vi "signal_generation_0.vi"() -> ()   [LabVIEW 2016]
uses:
  controls/State.ctl
  <vilib>/Utility/error.llb/DialogType.ctl
  <vilib>/DAQmx/write.llb/DAQmx Write (Analog Wfm 1Chan NSamp).vi
  <vilib>/DAQmx/write.llb/DAQmx Write (Analog DBL 1Chan 1Samp).vi
  <vilib>/DAQmx/read.llb/DAQmx Read (Analog 1D Wfm NChan NSamp).vi
  <vilib>/DAQmx/create/channels.llb/DAQmx Create Channel (AO-Voltage-Basic).vi
  <vilib>/DAQmx/create/channels.llb/DAQmx Create Channel (AI-Voltage-Basic).vi
  <vilib>/DAQmx/configure/timing.llb/DAQmx Timing (Sample Clock).vi
  <vilib>/DAQmx/miscellaneous.llb/DAQmx Fill In Error Info.vi
  <resource>/objmgr/daqmx.rc
  <vilib>/measure/NI_MABase.lvlib
panel:
  out "Waveform Graph 2":waveform(dbl)[](graph)=[{"t0"=timestamp(3594732894.3389087 s since 1904-01-01), "dt"=0.001, "Y"=array[1000 elements], "attributes"=variant("NI_ChannelName"=variant(string "DAQ_6363/ai0"), "NI_UnitDescription"=variant(string "Volts"))}]
  in  "DAQ channel 3 In":tag="DAQ_6363/ai0"
  out "error out":errorcluster
  in  "Number of Samples":i32=1000
  in  "Samples per Period":dbl=100.0
  in  "DAQ channel 2 In":tag="DAQ_6363/ao1"
  in  "DAQ channel 1 In":tag="DAQ_6363/ao0"
  in  "Error In (no error)":errorcluster
  in  "Exit Button":bool
  out "Status":string="Off"
  in  "TMA Voltage On/Off":bool
  in  "Sawtooth Signal On/Off":bool
  out "Waveform Graph":waveform(dbl)(graph)={"t0"=timestamp(0 s since 1904-01-01), "dt"=0.001, "Y"=array[1000 elements]}
  in  "TMA Voltage":dbl=2.0 min=-10.0 max=10.0
  in  "Period (ms)":dbl=100.0 min=0.01
  in  "Amplitude (V)":dbl=2.0 min=0.0 max=30.0
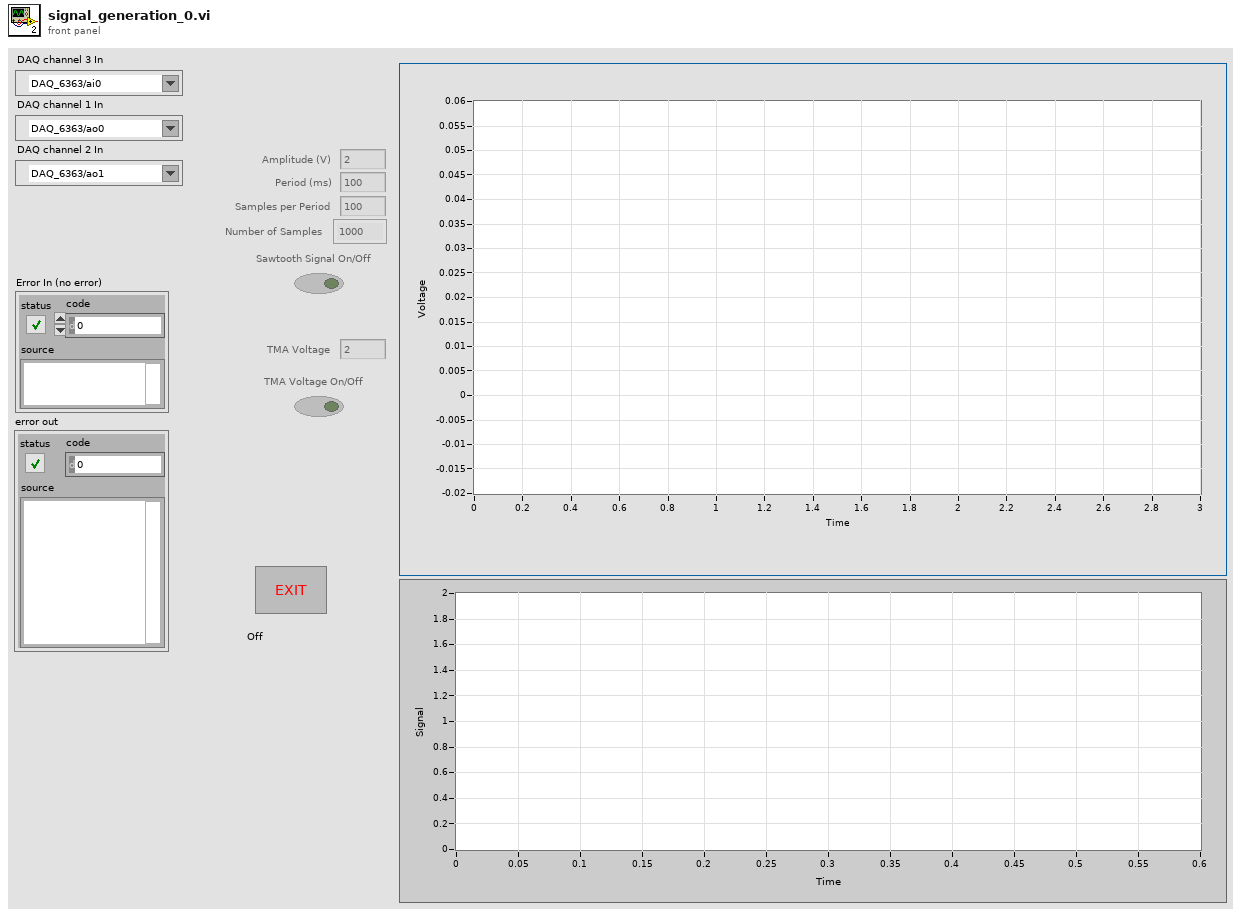
[diagram p1: front panel]
types:
  T1 = typedef "State.ctl" = enum16{"Init", "Idle", "Shutdown"}
  T2 = enum16{"Sine Wave", "Triangle Wave", "Square Wave", "Sawtooth Wave"}
  T3 = typedef "DialogType.ctl" = u16
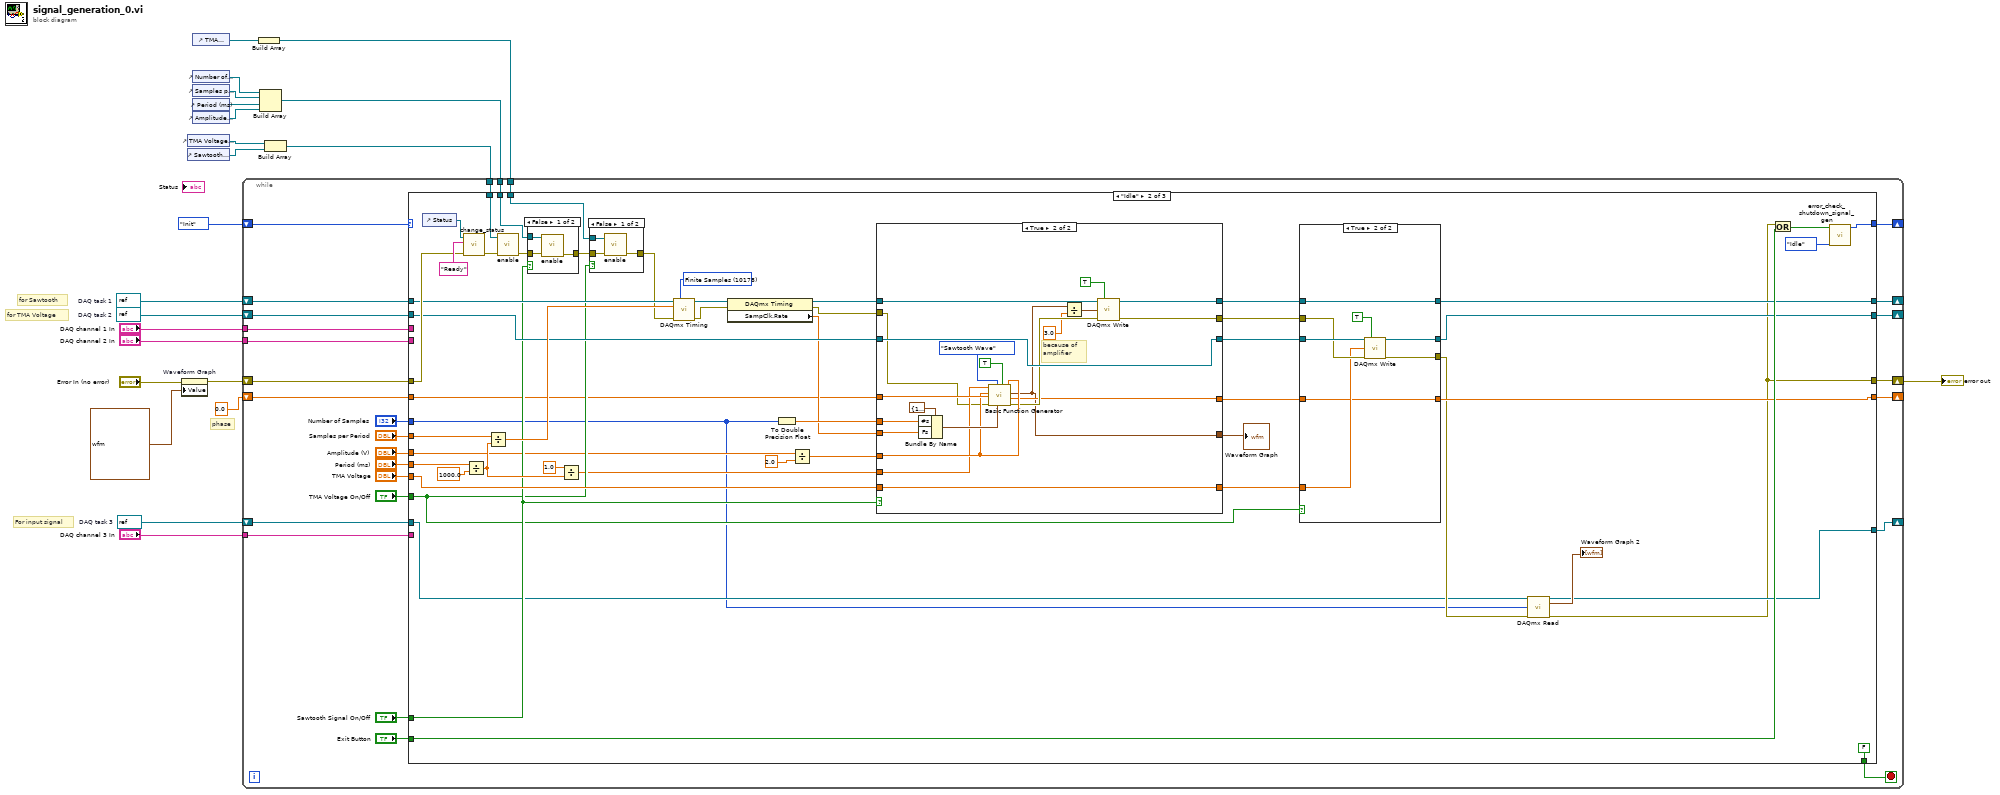
[diagram p0: block diagram]
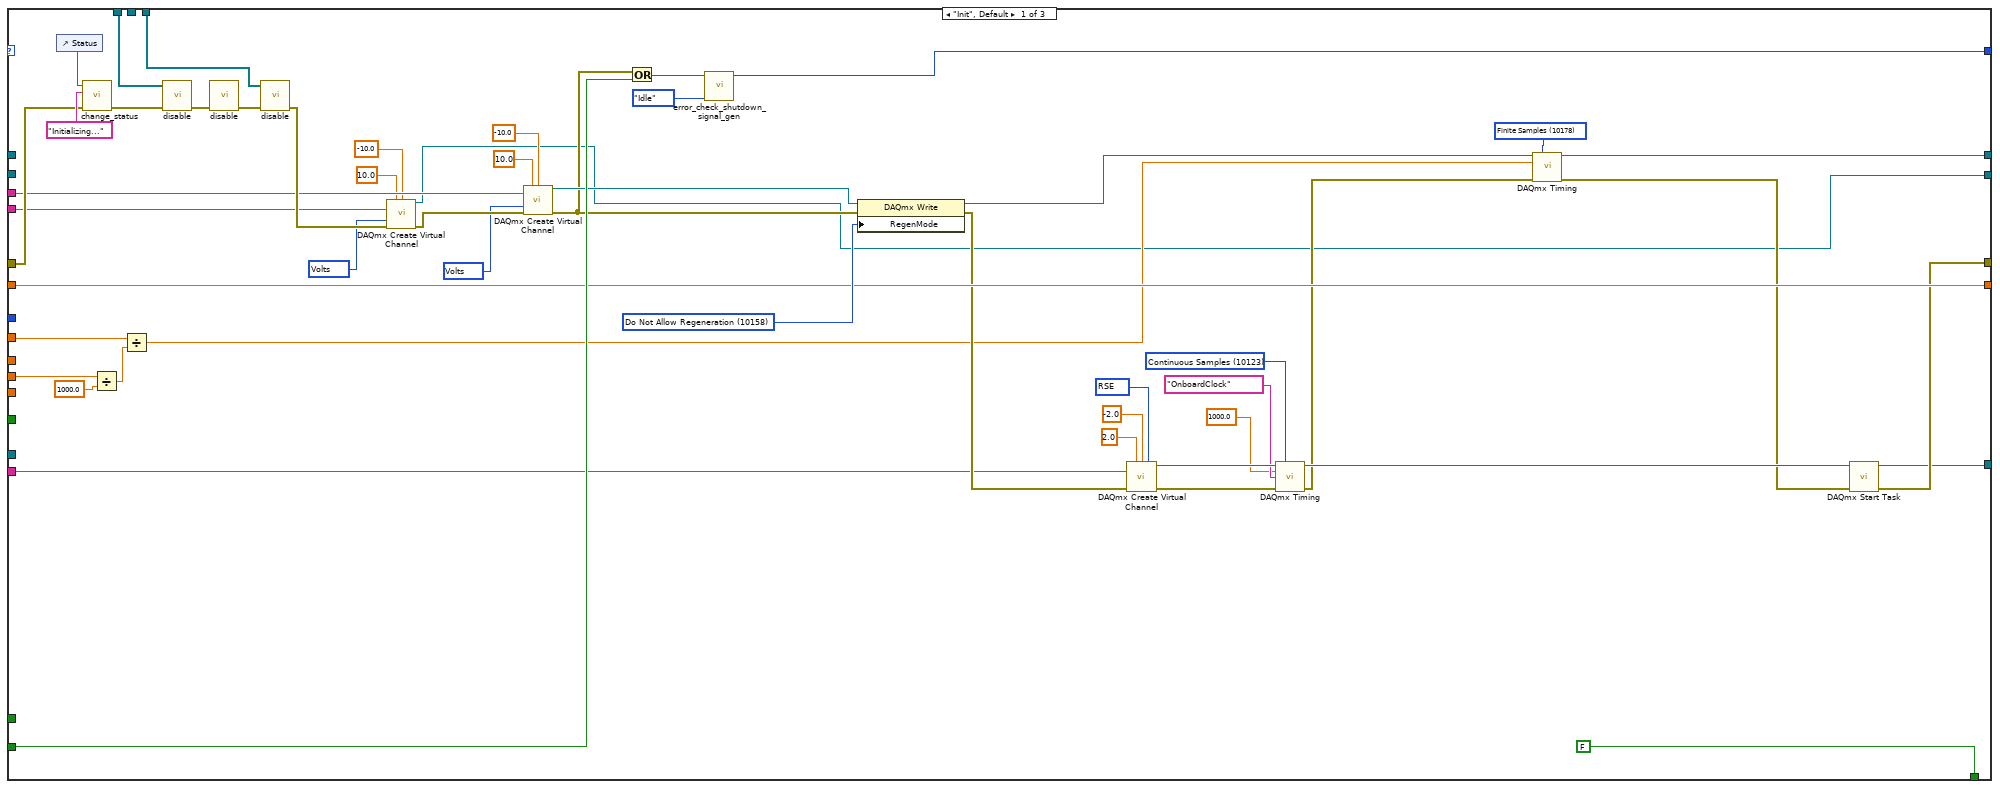
[diagram p2: hidden frame]
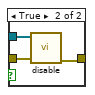
[diagram p3: hidden frame]
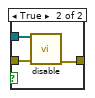
[diagram p4: hidden frame]
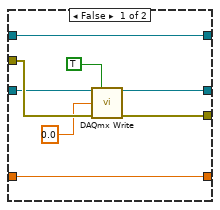
[diagram p5: hidden frame]
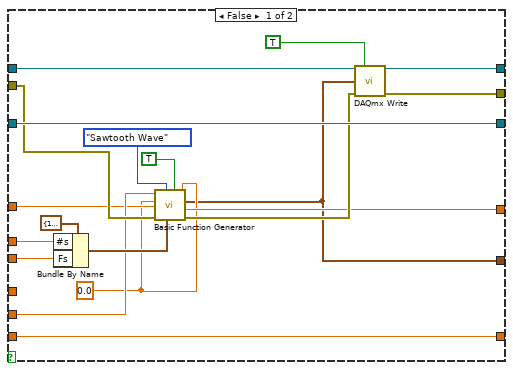
[diagram p6: hidden frame]
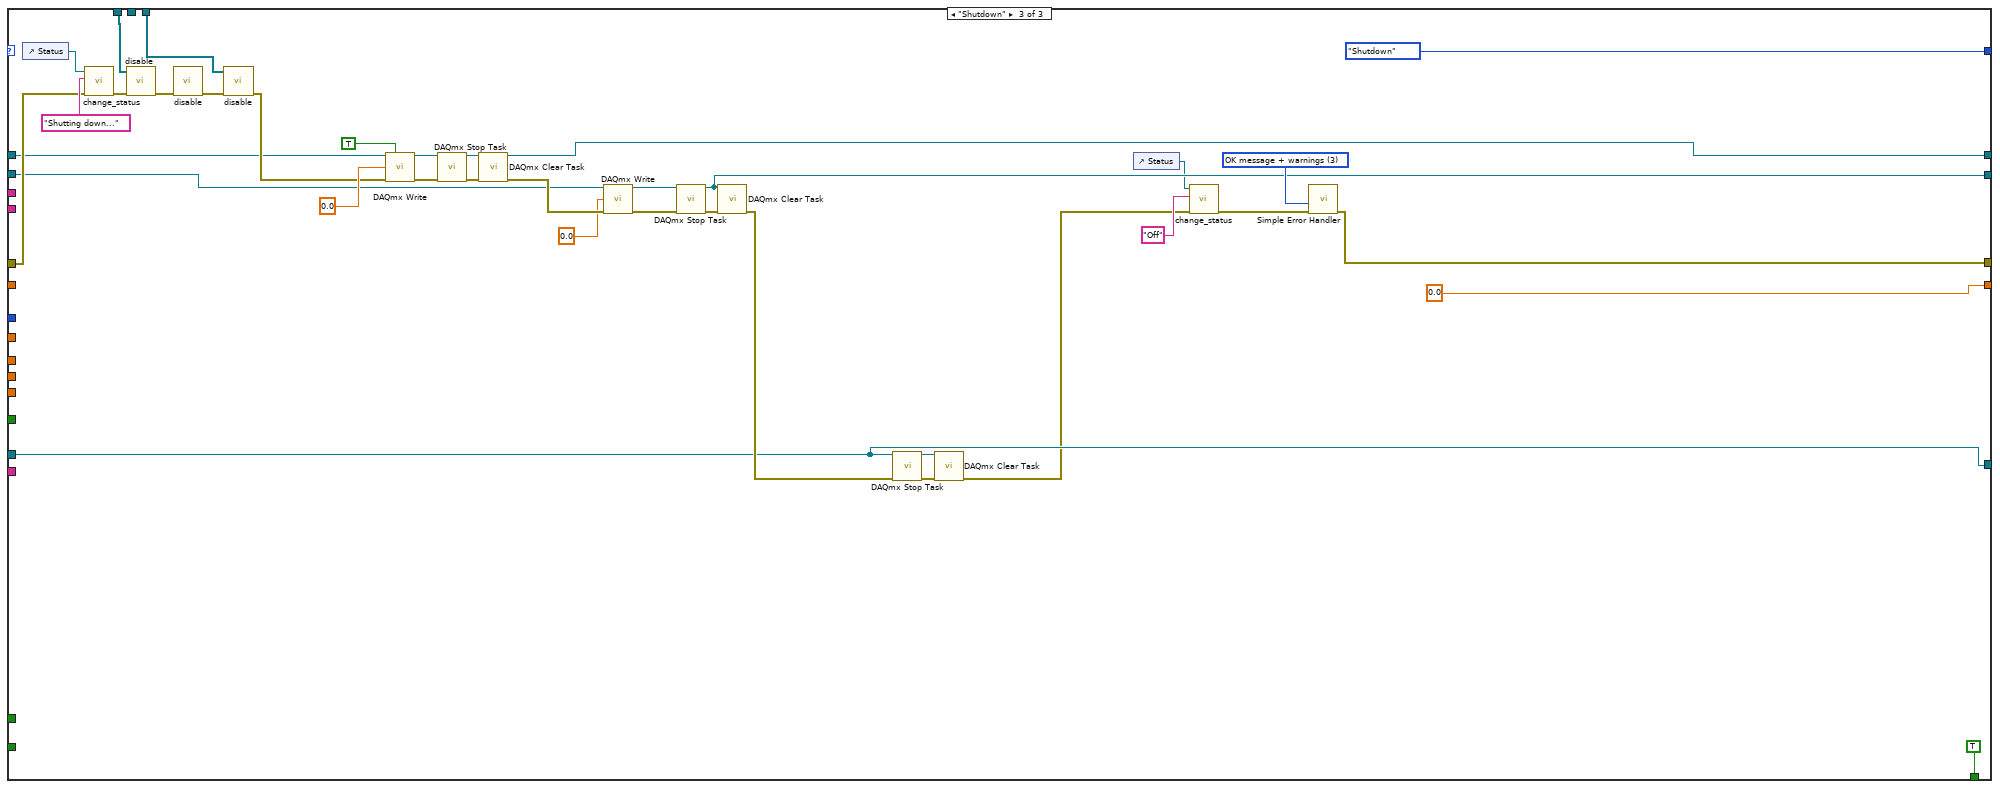
[diagram p7: hidden frame]
diagram:
  w1 = refnum<k21> refnum  # DAQ task 3
  w14 = refnum<k21> refnum  # DAQ task 1
  w13 = refnum<k21> refnum  # DAQ task 2
  # "For input signal"
  # "phase"
  # "for TMA Voltage"
  # "for Sawtooth"
  n1 = property on="Waveform Graph" class="WFGraph (strict)"(error in="Error In (no error)", "Value"=waveform(dbl) {"t0"=timestamp(0 s since 1904-01-01), "dt"=1.0, "Y"=[]} ("Waveform Graph")) -> (error out=w17:errorcluster)  [unwired: 1 in, 1 out]
  n2 = control-ref of="TMA Voltage On/Off"() -> (w21:refnum<vi>)
  n3 = control-ref of="Sawtooth Signal On/Off"() -> (w20:refnum<vi>)
  n4 = control-ref of="TMA Voltage"() -> (w3:refnum<vi>)
  n5 = control-ref of="Number of Samples"() -> (w7:refnum<vi>)
  n6 = control-ref of="Samples per Period"() -> (w6:refnum<vi>)
  n7 = control-ref of="Period (ms)"() -> (w5:refnum<vi>)
  n8 = control-ref of="Amplitude (V)"() -> (w4:refnum<vi>)
  n9 = Build Array(w3) -> (w9:refnum<vi>[])
  n10 = Build Array(w7, w6, w5, w4) -> (w10:refnum<vi>[])
  n11 = Build Array(w21, w20) -> (w19:refnum<vi>[])
  n12 = while {
    shift-right: [w35] -> _
    shift-left: State."Init" -> [w49]
    tunnel: w19 -> [w48]
    shift-right: [w34] -> w8
    shift-left: w17 -> [w42]
    tunnel: "DAQ channel 1 In" -> [w41]
    tunnel: "DAQ channel 2 In" -> [w40]
    shift-right: [w37] -> _
    shift-left: w14 -> [w39]
    shift-right: [w36] -> _
    shift-left: w13 -> [w38]
    shift-right: [w30] -> _
    shift-left: 0.0 -> [w31]
    tunnel: w10 -> [w29]
    tunnel: w9 -> [w28]
    tunnel: "DAQ channel 3 In" -> [w25]
    shift-right: [w24] -> _
    shift-left: w1 -> [w23]
    stop <- w27 stop-if-true
    n13 = case shown="\"Idle\"" w49 {
      tunnel: w48 -> [w97 w153 w251]
      tunnel: "Amplitude (V)" -> [_ w117 _]
      tunnel: "Period (ms)" -> [w56 w145 _]
      tunnel: "TMA Voltage" -> [_ w133 _]
      tunnel: "TMA Voltage On/Off" -> [_ w121 _]
      tunnel: "Sawtooth Signal On/Off" -> [_ w122 _]
      tunnel: "Exit Button" -> [w89 w129 _]
      tunnel: w42 -> [w96 w148 w254]
      tunnel: w41 -> [w93 _ _]
      tunnel: w40 -> [w94 _ _]
      tunnel: [w57 w127 w231] -> w37
      tunnel: [w50 w126 w232] -> w36
      tunnel: w39 -> [_ w147 w240]
      tunnel: w38 -> [_ w135 w235]
      tunnel: [w86 w128 State."Shutdown" ("State Out")] -> w35
      tunnel: [w63 w103 w233] -> w34
      tunnel: "Samples per Period" -> [w52 w101 _]
      tunnel: "Number of Samples" -> [_ w102 _]
      tunnel: w31 -> [w80 w111 _]
      tunnel: [w80 w109 0.0 ("phase out")] -> w30
      tunnel: w29 -> [_ w123 _]
      tunnel: w28 -> [w81 w120 w250]
      tunnel: [FALSE FALSE TRUE] -> w27
      tunnel: w25 -> [w73 _ _]
      tunnel: [w62 w104 w223] -> w24
      tunnel: w23 -> [_ w105 w223]
      frame "Init", Default {
        w61 = 10178 items=["Finite Samples"=10178, "Continuous Samples"=10123, "Hardware Timed Single Point"=12522] ("sample mode")
        w65 = 10123 items=["Finite Samples"=10178, "Continuous Samples"=10123, "Hardware Timed Single Point"=12522] ("sample mode")
        w70 = 10083 items=["Default"=-1, "RSE"=10083, "NRSE"=10078, "Differential"=10106, "Pseudodifferential"=12529] ("input terminal configuration")
        w84 = 10158 items=["Allow Regeneration"=10097, "Do Not Allow Regeneration"=10158] ("RegenMode")
        w90 = 10348 items=["Volts"=10348, "From Custom Scale"=10065] ("units")
        w91 = 10348 items=["Volts"=10348, "From Custom Scale"=10065] ("units")
        n14 = control-ref of="Status"() -> (w98:refnum<vi>)
        n15 = call "change_status.vi"("error in (no error)"=w96, "String"="Initializing...", "String in"=w98) -> ("error out"=w100:errorcluster)  [unwired: 8 in]
        n16 = Divide(x=w56, y=1000.0) -> (x/y=w54:dbl)
        n17 = Divide(x=w52, y=w54) -> (x/y=w53:dbl)
        n18 = call "disable.vi"("error in (no error)"=w100, "Array"=w97) -> ("error out"=w83:errorcluster)  [unwired: 9 in]
        n19 = call "disable.vi"("error in (no error)"=w83) -> ("error out"=w82:errorcluster)  [unwired: 10 in]
        n20 = call "disable.vi"("error in (no error)"=w82, "Array"=w81) -> ("error out"=w95:errorcluster)  [unwired: 9 in]
        n21 = call-poly <vilib>:"DAQmx Create Virtual Channel.vi"("maximum value"=10.0, "minimum value"=-10.0, "physical channels"=w94, "units"=w91, "error in"=w95) -> ("task out"=w50:refnum<k21>, "error out"=w92:errorcluster)  [unwired: 9 in]
        n22 = call-poly <vilib>:"DAQmx Create Virtual Channel.vi"("maximum value"=10.0, "minimum value"=-10.0, "physical channels"=w93, "units"=w90, "error in"=w92) -> ("task out"=w85:refnum<k21>, "error out"=w51:errorcluster)  [unwired: 9 in]
        n23 = Or(x=w51, y=w89) -> (x .or. y?=w88:bool)
        n24 = call "error_check_shutdown_signal_gen.vi"("State In"=State."Idle", "Boolean"=w88) -> ("State Out"=w86:T1)  [unwired: 9 in]
        n25 = property class="DAQmx Write"(reference=w85, error in=w51, "RegenMode"=w84) -> (reference out=w58:refnum<k21>, error out=w74:errorcluster)
        n26 = call-poly <vilib>:"DAQmx Create Virtual Channel.vi"("maximum value"=2.0, "minimum value"=-2.0, "input terminal configuration"=w70, "physical channels"=w73, "error in"=w74) -> ("task out"=w68:refnum<k21>, "error out"=w69:errorcluster)  [unwired: 9 in]
        n27 = call-poly <vilib>:"DAQmx Timing.vi"("task/channels in"=w68, "sample mode"=w65, "rate"=1000.0, "source"=tag "OnboardClock", "error in"=w69) -> ("task out"=w64:refnum<k21>, "error out"=w60:errorcluster)  [unwired: 9 in]
        n28 = call-poly <vilib>:"DAQmx Timing.vi"("task/channels in"=w58, "sample mode"=w61, "rate"=w53, "error in"=w60) -> ("task out"=w57:refnum<k21>, "error out"=w59:errorcluster)  [unwired: 10 in]
        n29 = call <vilib>:"DAQmx Start Task.vi"("task/channels in"=w64, "error in"=w59) -> ("task out"=w62:refnum<k21>, "error out"=w63:errorcluster)  [unwired: 12 in]
      }
      frame "Idle" {
        w146 = 10178 items=["Finite Samples"=10178, "Continuous Samples"=10123, "Hardware Timed Single Point"=12522] ("sample mode")
        n30 = control-ref of="Status"() -> (w150:refnum<vi>)
        n31 = call "change_status.vi"("error in (no error)"=w148, "String"="Ready", "String in"=w150) -> ("error out"=w152:errorcluster)  [unwired: 8 in]
        n32 = Divide(x=w145, y=1000.0) -> (x/y=w139:dbl)
        n33 = Divide(x=w101, y=w139) -> (x/y=w143:dbl)
        n34 = call "enable.vi"("error in (no error)"=w152, "Array"=w153) -> ("error out"=w151:errorcluster)  [unwired: 9 in]
        n35 = case shown="False" w122 {
          tunnel: w151 -> [w162 w165]
          tunnel: [w161 w164] -> w125
          tunnel: w123 -> [w160 w163]
          frame False {
            n36 = call "enable.vi"("error in (no error)"=w162, "Array"=w160) -> ("error out"=w161:errorcluster)  [unwired: 9 in]
          }
          frame True {
            n37 = call "disable.vi"("error in (no error)"=w165, "Array"=w163) -> ("error out"=w164:errorcluster)  [unwired: 9 in]
          }
        }
        n38 = Divide(x=1.0, y=w139) -> (x/y=w113:dbl)
        n39 = case shown="False" w121 {
          tunnel: w125 -> [w156 w159]
          tunnel: [w155 w158] -> w124
          tunnel: w120 -> [w154 w157]
          frame False {
            n40 = call "enable.vi"("error in (no error)"=w156, "Array"=w154) -> ("error out"=w155:errorcluster)  [unwired: 9 in]
          }
          frame True {
            n41 = call "disable.vi"("error in (no error)"=w159, "Array"=w157) -> ("error out"=w158:errorcluster)  [unwired: 9 in]
          }
        }
        n42 = call-poly <vilib>:"DAQmx Timing.vi"("task/channels in"=w147, "sample mode"=w146, "rate"=w143, "error in"=w124) -> ("task out"=w142:refnum<k21>, "error out"=w141:errorcluster)  [unwired: 10 in]
        n43 = property class="DAQmx Timing"(reference=w142, error in=w141) -> (reference out=w138:refnum<k21>, error out=w114:errorcluster, "SampClk.Rate"=w115:dbl)
        n44 = To Double Precision Float(number=w102) -> (double precision float=w116:dbl)
        n45 = Divide(x=w117, y=2.0) -> (x/y=w112:dbl)
        n46 = case shown="True" w122 {
          tunnel: w138 -> [w198 w221]
          tunnel: [w197 w218] -> w137
          tunnel: [w196 w217] -> w136
          tunnel: w135 -> [w200 w220]
          tunnel: [w200 w220] -> w134
          tunnel: w133 -> [w199 w219]
          tunnel: [w199 w219] -> w132
          tunnel: w116 -> [w193 w210]
          tunnel: w115 -> [w192 w209]
          tunnel: w114 -> [w188 w206]
          tunnel: w113 -> [w186 w207]
          tunnel: w112 -> [_ w208]
          tunnel: w111 -> [w185 w211]
          tunnel: [w184 w204] -> w110
          tunnel: [w182 w202] -> w108
          frame False {
            w183 = 0.0
            n47 = Bundle By Name(cluster=cluster{"Fs":dbl, "#s":dbl} {"Fs"=1000.0, "#s"=1000.0} ("sampling info"), "#s"=w193, "Fs"=w192) -> (w191:cluster{"Fs":dbl, "#s":dbl})
            n48 = call <vilib>:"Basic Function Generator.vi"("offset"=w183, "reset signal"=TRUE, "sampling info"=w191, "signal type"=T2."Sawtooth Wave", "error in (no error)"=w188, "phase"=w185, "amplitude"=w183, "frequency"=w186) -> ("error out"=w187:errorcluster, "phase out"=w184:dbl, "signal out"=w182:waveform(dbl))  [unwired: 1 in]
            n49 = call-poly <vilib>:"DAQmx Write.vi"("task/channels in"=w198, "auto start"=TRUE, "data"=w182, "error in"=w187) -> ("task out"=w197:refnum<k21>, "error out"=w196:errorcluster)  [unwired: 9 in, 1 out]
          }
          frame True {
            # "because of \namplifier"
            n50 = Bundle By Name(cluster=cluster{"Fs":dbl, "#s":dbl} {"Fs"=1000.0, "#s"=1000.0} ("sampling info"), "#s"=w210, "Fs"=w209) -> (w214:cluster{"Fs":dbl, "#s":dbl})
            n51 = call <vilib>:"Basic Function Generator.vi"("offset"=w208, "reset signal"=TRUE, "sampling info"=w214, "signal type"=T2."Sawtooth Wave", "error in (no error)"=w206, "phase"=w211, "amplitude"=w208, "frequency"=w207) -> ("error out"=w205:errorcluster, "phase out"=w204:dbl, "signal out"=w202:waveform(dbl))  [unwired: 1 in]
            n52 = Divide(x=w202, y=3.0) -> (x/y=w201:waveform(dbl))
            n53 = call-poly <vilib>:"DAQmx Write.vi"("task/channels in"=w221, "auto start"=TRUE, "data"=w201, "error in"=w205) -> ("task out"=w218:refnum<k21>, "error out"=w217:errorcluster)  [unwired: 9 in, 1 out]
          }
        }
        "Waveform Graph" <- w108
        n54 = case shown="True" w121 {
          tunnel: w137 -> [w173 w181]
          tunnel: w136 -> [w171 w178]
          tunnel: w134 -> [w170 w180]
          tunnel: [w173 w181] -> w127
          tunnel: [w169 w179] -> w126
          tunnel: [w172 w177] -> w106
          tunnel: w132 -> [_ w176]
          tunnel: w110 -> [w166 w174]
          tunnel: [w166 w174] -> w109
          frame False {
            n55 = call-poly <vilib>:"DAQmx Write.vi"("task/channels in"=w170, "auto start"=TRUE, "data"=0.0, "error in"=w171) -> ("task out"=w169:refnum<k21>, "error out"=w172:errorcluster)  [unwired: 9 in, 1 out]
          }
          frame True {
            n56 = call-poly <vilib>:"DAQmx Write.vi"("task/channels in"=w180, "auto start"=TRUE, "data"=w176, "error in"=w178) -> ("task out"=w179:refnum<k21>, "error out"=w177:errorcluster)  [unwired: 9 in, 1 out]
          }
        }
        n57 = call-poly <vilib>:"DAQmx Read.vi"("task/channels in"=w105, "number of samples per channel"=w102, "error in"=w106) -> ("task out"=w104:refnum<k21>, "data"=→"Waveform Graph 2":waveform(dbl)[], "error out"=w103:errorcluster)  [unwired: 10 in]
        n58 = Or(x=w103, y=w129) -> (x .or. y?=w131:bool)
        n59 = call "error_check_shutdown_signal_gen.vi"("State In"=State."Idle", "Boolean"=w131) -> ("State Out"=w128:T1)  [unwired: 9 in]
      }
      frame "Shutdown" {
        w246 = T3 3 items=["no dialog", "OK message", "continue or stop message", "OK message + warnings", "continue/stop + warnings"] ("type of dialog (OK msg:1)")
        n60 = control-ref of="Status"() -> (w257:refnum<vi>)
        n61 = call "change_status.vi"("error in (no error)"=w254, "String"="Shutting down...", "String in"=w257) -> ("error out"=w255:errorcluster)  [unwired: 8 in]
        n62 = call "disable.vi"("error in (no error)"=w255, "Array"=w251) -> ("error out"=w253:errorcluster)  [unwired: 9 in]
        n63 = call "disable.vi"("error in (no error)"=w253) -> ("error out"=w252:errorcluster)  [unwired: 10 in]
        n64 = call "disable.vi"("error in (no error)"=w252, "Array"=w250) -> ("error out"=w241:errorcluster)  [unwired: 9 in]
        n65 = call-poly <vilib>:"DAQmx Write.vi"("task/channels in"=w240, "auto start"=TRUE, "data"=0.0, "error in"=w241) -> ("task out"=w242:refnum<k21>, "error out"=w243:errorcluster)  [unwired: 9 in, 1 out]
        n66 = call <vilib>:"DAQmx Stop Task.vi"("task/channels in"=w242, "error in"=w243) -> ("task out"=w231:refnum<k21>, "error out"=w247:errorcluster)  [unwired: 12 in]
        n67 = call <vilib>:"DAQmx Clear Task.vi"("task in"=w231, "error in"=w247) -> ("error out"=w239:errorcluster)  [unwired: 13 in]
        n68 = call-poly <vilib>:"DAQmx Write.vi"("task/channels in"=w235, "data"=0.0, "error in"=w239) -> ("task out"=w237:refnum<k21>, "error out"=w238:errorcluster)  [unwired: 10 in, 1 out]
        n69 = call <vilib>:"DAQmx Stop Task.vi"("task/channels in"=w237, "error in"=w238) -> ("task out"=w232:refnum<k21>, "error out"=w245:errorcluster)  [unwired: 12 in]
        n70 = call <vilib>:"DAQmx Clear Task.vi"("task in"=w232, "error in"=w245) -> ("error out"=w224:errorcluster)  [unwired: 13 in]
        n71 = call <vilib>:"DAQmx Stop Task.vi"("task/channels in"=w223, "error in"=w224) -> ("task out"=w225:refnum<k21>, "error out"=w226:errorcluster)  [unwired: 12 in]
        n72 = call <vilib>:"DAQmx Clear Task.vi"("task in"=w225, "error in"=w226) -> ("error out"=w222:errorcluster)  [unwired: 13 in]
        n73 = control-ref of="Status"() -> (w228:refnum<vi>)
        n74 = call "change_status.vi"("error in (no error)"=w222, "String"="Off", "String in"=w228) -> ("error out"=w229:errorcluster)  [unwired: 8 in]
        n75 = call <vilib>:"Simple Error Handler.vi"("type of dialog (OK msg:1)"=w246, "error in (no error)"=w229) -> ("error out"=w233:errorcluster)  [unwired: 3 in, 4 out]
      }
    }
  }
  "error out" <- w8
